vi "Add to Project.vi"(8 "error in (no error)":errorcluster, 11 "Coupled Message Rescripter in":refnum<class "Coupled Message Rescripter.lvclass">) -> (0 "error out":errorcluster, 3 "Coupled Message Rescripter out":refnum<class "Coupled Message Rescripter.lvclass">)   [LabVIEW 2020, in "Message Rescripter.lvlib" / "Coupled Message Rescripter.lvclass"]
uses:
  Coupled Message Rescripter.lvclass
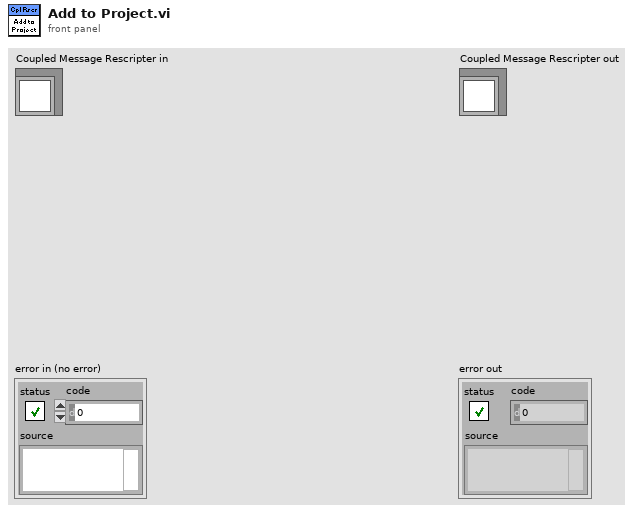
[diagram p1: front panel]
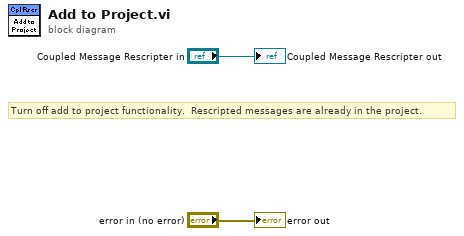
[diagram p0: block diagram]
diagram:
  # "Turn off add to project functionality.  Rescripted messages are already in the project."
  "error out" <- "error in (no error)"
  "Coupled Message Rescripter out" <- "Coupled Message Rescripter in"
